vi "Read Duration per Period.vi"(11 "User Interface in":refnum<class "User Interface.lvclass">) -> (2 "Duration per Period":refnum<vi>, 3 "User Interface out":refnum<class "User Interface.lvclass">)   [LabVIEW 2016, in "User Interface.lvlib" / "User Interface.lvclass"]
uses:
  User Interface.lvclass
  User Interface.lvclass/User Interface.ctl
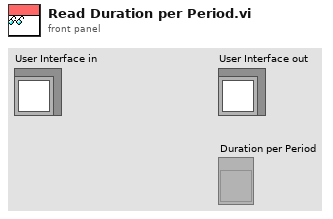
[diagram p1: front panel]
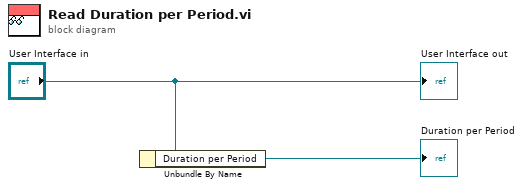
[diagram p0: block diagram]
diagram:
  n1 = Unbundle By Name("User Interface in") -> ("Duration per Period"=→"Duration per Period":refnum<vi>)
  "User Interface out" <- "User Interface in"
